vi "Stream Compress Splitter.vi"(9 "Array lengh":i32, 10 "Ending edges":i32[](array[numeric]), 11 "Starting edges":i32[](array[numeric])) -> (3 "Segments":T1[](array[typedef]))   [LabVIEW 2016]
uses:
  Stream Segment.ctl
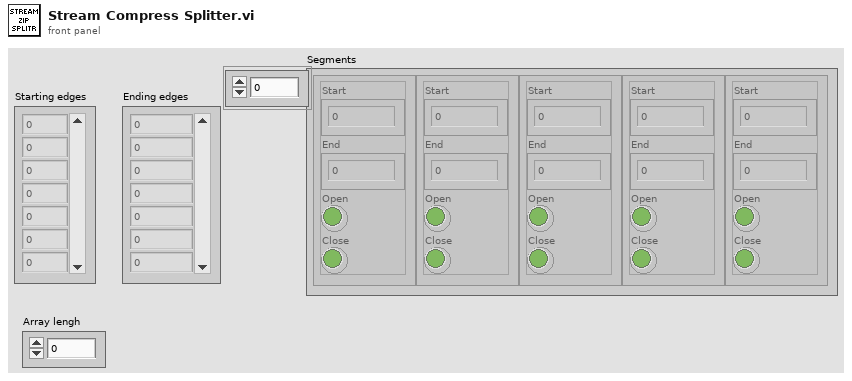
[diagram p1: front panel]
types:
  T1 = typedef "Stream Segment.ctl" = cluster{"Start":i32, "End":i32, "Open":bool, "Close":bool}
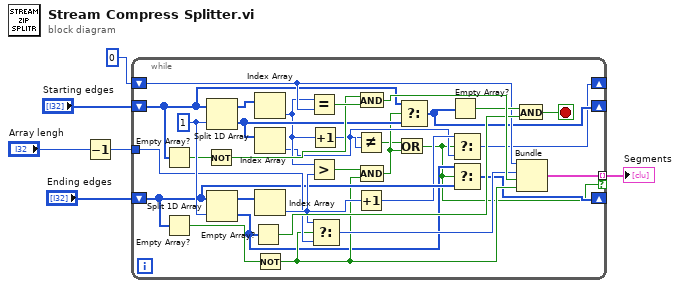
[diagram p0: block diagram]
diagram:
  n1 = Decrement(x="Array lengh") -> (x-1=w1:i32)
  n2 = while {
    shift-right: [w15] -> _
    shift-left: "Starting edges" -> [w14]
    shift-right: [w10] -> _
    shift-left: "Ending edges" -> [w21]
    shift-right: [w12] -> _
    shift-left: 0 -> [w29]
    tunnel: w1 -> [w23]
    tunnel: [w30] -> w2 mode=indexing if=w7
    stop <- w31 stop-if-true
    w36 = 1 ("index")
    n3 = Empty Array?(array=w14) -> (empty?=w35:bool)
    n4 = Empty Array?(array=w21) -> (empty?=w28:bool)
    n5 = Not(x=w35) -> (.not. x?=w25:bool)
    n6 = Split 1D Array(array=w14, index=w36) -> (first subarray=w38:i32[], second subarray=w19:i32[])
    n7 = Split 1D Array(array=w21, index=w36) -> (first subarray=w37:i32[], second subarray=w16:i32[])
    n8 = Empty Array?(array=w16) -> (empty?=w32:bool)
    n9 = Index Array(array=w38) -> (element=w18:i32)  [unwired: 1 in]
    n10 = Index Array(array=w19) -> (element=w11:i32)  [unwired: 1 in]
    n11 = Index Array(array=w37) -> (element=w24:i32)  [unwired: 1 in]
    n12 = Not(x=w28) -> (.not. x?=w20:bool)
    n13 = Equal?(x=w18, y=w29) -> (x = y?=w27:bool)
    n14 = Greater?(x=w18, y=w24) -> (0:w26:bool)
    n15 = Increment(x=w18) -> (x+1=w17:i32)
    n16 = Select(t=w24, s=w20, f=w23) -> (s? t:f=w22:i32)
    n17 = Not Equal?(x=w11, y=w17) -> (x != y?=w8:bool)
    n18 = Increment(x=w24) -> (x+1=w13:i32)
    n19 = And(x=w25, y=w27) -> (x .and. y?=w34:bool)
    n20 = Compound Arithmetic op=AND(w26, w20) -> (w9:bool)
    n21 = Or(x=w8, y=w9) -> (x .or. y?=w7:bool)
    n22 = Select(t=w14, s=w9, f=w19) -> (s? t:f=w15:i32[])
    n23 = Empty Array?(array=w15) -> (empty?=w33:bool)
    n24 = Select(t=w13, s=w7, f=w11) -> (s? t:f=w12:i32)
    n25 = Select(t=w16, s=w7, f=w21) -> (s? t:f=w10:i32[])
    n26 = And(x=w33, y=w32) -> (x .and. y?=w31:bool)
    n27 = Bundle(w29, "Numeric"=w22, w34, w20) -> (w30:cluster{i32, "Numeric":i32, bool, bool})  [unwired: 1 in]
  }
  "Segments" <- w2
